vi "OPC UA Server_String.vi"() -> ()   [LabVIEW 2017]
uses:
  <vilib>/OPCUA/controls/Data Type.ctl
  <vilib>/OPCUA/NI OPC UA Server.lvlib
panel:
  in  "stop":bool
  out "error out":errorcluster
  out "item node ID":string
  out "server endpoint URL":string
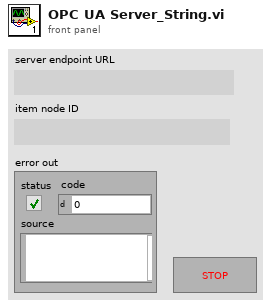
[diagram p1: front panel]
types:
  T1 = typedef "Data Type.ctl" = u16
  T2 = cluster{"name":string, "data type":T1, "access level":u16, "description":string}
  T3 = typedef "OPC UA Server Refnum.ctl" = refnum<k21>
  T4 = typedef "NodeId.ctl" = string
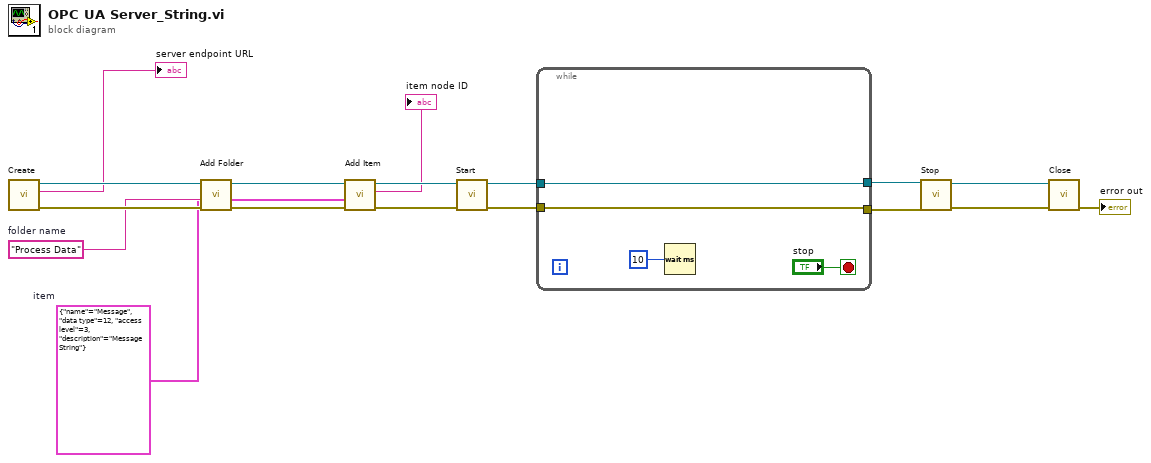
[diagram p0: block diagram]
diagram:
  w9 = T2 {"name"="Message", "data type"=12, "access level"=3, "description"="Message String"}  # item
  w10 = "Process Data"  # folder name
  n1 = call <vilib>:"Create.vi"() -> ("error out"=w14:errorcluster, "server endpoint URL"=→"server endpoint URL":string, "OPC UA server refnum out"=w17:T3)  [unwired: 9 in]
  n2 = call <vilib>:"Add Folder.vi"("error in (no error)"=w14, "folder name"=w10, "OPC UA server refnum in"=w17) -> ("error out"=w13:errorcluster, "OPC UA server refnum out"=w16:T3)  [unwired: 5 in, 1 out]
  n3 = call <vilib>:"Add Item.vi"("error in (no error)"=w13, "item"=w9, "OPC UA server refnum in"=w16) -> ("error out"=w12:errorcluster, "item node ID"=→"item node ID":T4, "OPC UA server refnum out"=w15:T3)  [unwired: 4 in, 1 out]
  n4 = call <vilib>:"Start.vi"("error in (no error)"=w12, "OPC UA server refnum in"=w15) -> ("error out"=w6:errorcluster, "OPC UA server refnum out"=w7:T3)  [unwired: 7 in, 1 out]
  n5 = while {
    tunnel: [w21] -> w4
    tunnel: w7 -> [w21]
    tunnel: [w20] -> w5
    tunnel: w6 -> [w20]
    stop <- "stop" stop-if-true
    n6 = Wait (ms)(milliseconds to wait=u32 10) -> ()  [unwired: 1 out]
  }
  n7 = call <vilib>:"Stop.vi"("error in (no error)"=w5, "OPC UA server refnum in"=w4) -> ("error out"=w2:errorcluster, "OPC UA server refnum out"=w3:T3)  [unwired: 8 in]
  n8 = call <vilib>:"Close.vi"("error in (no error)"=w2, "OPC UA server refnum in"=w3) -> ("error out"=→"error out":errorcluster)  [unwired: 9 in]
